vi "TC_to_DSC.vi"(6 "AVS names":T1={"AVS Name 0"="3K", "AVS Name 1"="Still", "AVS Name 2"="50 mK", "AVS Name 3"="MC", "AVS Name 4"="MC", "AVS Name 5"="", "AVS Name 6"="", "AVS Name 7"="", "AVS Name 8"="", "AVS Name 9"=""}, 7 "AVS Type":T2(ring)=enum."CF_Z_Bridge", 8 "Array":refnum<vi>[](array[refnum]), 9 "I":dbl[](array[numeric]), 10 "T":dbl[](array[numeric]), 11 "R":dbl[](array[numeric])) -> ()   [LabVIEW 2013]
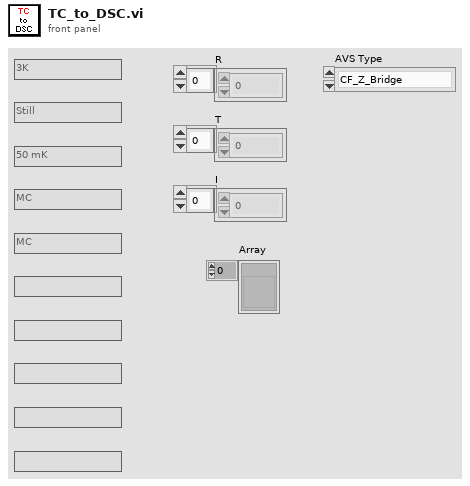
[diagram p1: front panel]
types:
  T1 = cluster{"AVS Name 0":string, "AVS Name 1":string, "AVS Name 2":string, "AVS Name 3":string, "AVS Name 4":string, "AVS Name 5":string, "AVS Name 6":string, "AVS Name 7":string, "AVS Name 8":string, "AVS Name 9":string}
  T2 = enum16{"CF", "CF_Z_Bridge", "MNK", "MNK_Z_Bridge"}
  T3 = cluster{"[0]":string, "[1]":string, "[2]":string, "[3]":string, "[4]":string, "[5]":string, "[6]":string, "[7]":string, "[8]":string, "[9]":string}
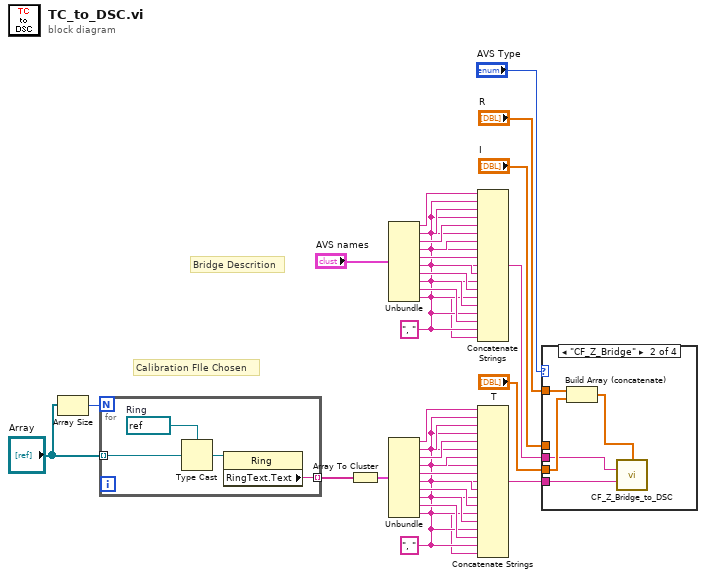
[diagram p0: block diagram]
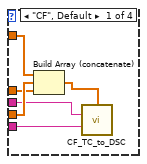
[diagram p2: hidden frame]
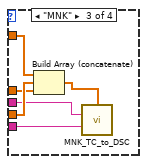
[diagram p3: hidden frame]
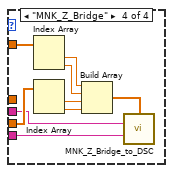
[diagram p4: hidden frame]
diagram:
  w5 = ", " ("string")
  w19 = ", " ("string")
  # "Bridge Descrition"
  # "Calibration FIle Chosen"
  n1 = Array Size(array="Array") -> (size(s)=w16:i32)
  n2 = for {
    N: w16 -> [_]
    tunnel: "Array" -> [w37] mode=indexing
    tunnel: [w34] -> w15 mode=indexing
    w36 = refnum<vi> refnum  # Ring
    n3 = Type Cast(type=w36, x=w37) -> (*(type *) &x=w35:refnum<vi>)
    n4 = property class="Ring"(reference=w35) -> ("RingText.Text"=w34:string)  [unwired: 1 in, 2 out]
  }
  n5 = Array To Cluster(array=w15) -> (cluster=w3:T3)
  n6 = Unbundle("AVS names") -> ("AVS Name 0"=w28:string, "AVS Name 1"=w27:string, "AVS Name 2"=w26:string, "AVS Name 3"=w25:string, "AVS Name 4"=w24:string, "AVS Name 5"=w23:string, "AVS Name 6"=w22:string, "AVS Name 7"=w21:string, "AVS Name 8"=w20:string, "AVS Name 9"=w18:string)
  n7 = Unbundle(w3) -> ("[0]"=w14:string, "[1]"=w13:string, "[2]"=w12:string, "[3]"=w11:string, "[4]"=w10:string, "[5]"=w9:string, "[6]"=w8:string, "[7]"=w7:string, "[8]"=w6:string, "[9]"=w4:string)
  n8 = Concatenate Strings(w28, w19, w27, w19, w26, w19, w25, w19, w24, w19, w23, w19, w22, w19, w21, w19, w20, w19, w18) -> (w17:string)
  n9 = Concatenate Strings(w14, w5, w13, w5, w12, w5, w11, w5, w10, w5, w9, w5, w8, w5, w7, w5, w6, w5, w4) -> (w1:string)
  n10 = case shown="\"CF_Z_Bridge\"" "AVS Type" {
    tunnel: "R" -> [w43 w48 w54 w62]
    tunnel: "T" -> [w42 w47 w53 w63]
    tunnel: "I" -> [w41 _ w52 _]
    tunnel: w17 -> [w39 w45 w49 w56]
    tunnel: w1 -> [w38 w44 w50 w55]
    frame "CF", Default {
      n11 = Build Array (concatenate)(w43, w42, w41) -> (w40:dbl[])
      n12 = call "CF_TC_to_DSC.vi"("dbl"=w40, "String In"=w39, "String In 2"=w38) -> ()  [unwired: 12 in, 1 out]
    }
    frame "CF_Z_Bridge" {
      n13 = Build Array (concatenate)(w48, w47) -> (w46:dbl[])
      n14 = call "CF_Z_Bridge_to_DSC.vi"("dbl"=w46, "String In"=w45, "String In 2"=w44) -> ()  [unwired: 12 in, 1 out]
    }
    frame "MNK" {
      n15 = Build Array (concatenate)(w54, w53, w52) -> (w51:dbl[])
      n16 = call "MNK_TC_to_DSC.vi"("dbl"=w51, "String In"=w49, "String In 2"=w50) -> ()  [unwired: 12 in, 1 out]
    }
    frame "MNK_Z_Bridge" {
      n17 = Index Array(array=w62) -> (element #1=w61:dbl, element #2=w60:dbl)  [unwired: 2 in]
      n18 = Index Array(array=w63) -> (element #1=w59:dbl, element #2=w58:dbl)  [unwired: 2 in]
      n19 = Build Array(w61, w60, w59, w58) -> (w57:dbl[])
      n20 = call "MNK_Z_Bridge_to_DSC.vi"("dbl"=w57, "String In"=w56, "String In 2"=w55) -> ()  [unwired: 13 in]
    }
  }
